vi "Write to File Core.vi"(8 "error in":errorcluster, 10 "File Ref":refnum<file>, 11 "Exe Write CRD RDs in":refnum<class "Exe Write CRD RDs.lvclass">) -> (0 "error out":errorcluster, 3 "Exe Write CRD RDs out":refnum<class "Exe Write CRD RDs.lvclass">)   [LabVIEW 2014, in "Controller.lvlib" / "Exe Write CRD RDs.lvclass"]
uses:
  Exe Write CRD RDs.lvclass
  reusable/Data/Data.lvclass
  Instr Exe Write to File/Instr Exe Write to File.lvclass/Instr Exe Write to File.ctl
  reusable/CRDS/Data/Main/CRDS Data.lvclass
  reusable/CRDS/Data/Cell/CRDS Cell Data.lvclass/CRDS Cell Data.ctl
  reusable/CRDS/Data/Cell/Read Laser Data.vi
  Instr Exe Write to File/Read MAP DVR.vi
  Instr Exe Write to File/Read DataObj.vi
  reusable/Data/Read measTime.vi
  reusable/CRDS/Data/Main/Read CellData.vi
  reusable/CRDS/Data/Cell/CRDS Cell Data.lvclass
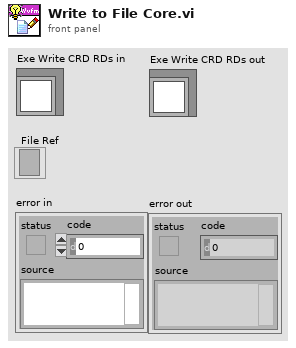
[diagram p1: front panel]
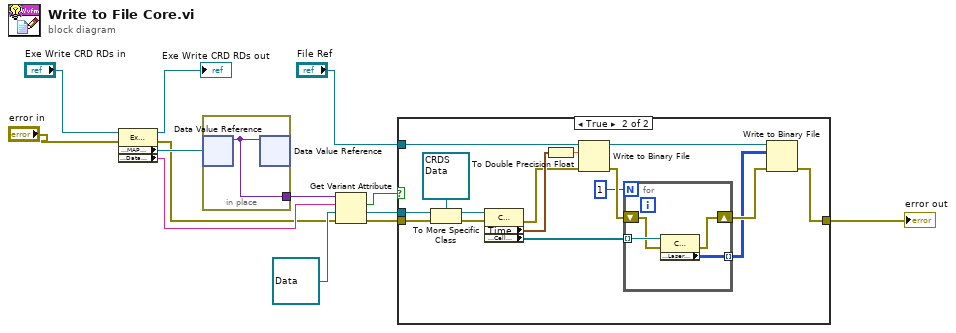
[diagram p0: block diagram]
diagram:
  n1 = property class="Exe Write CRD RDs"(reference="Exe Write CRD RDs in", error in="error in") -> (reference out=→"Exe Write CRD RDs out":refnum<class "Exe Write CRD RDs.lvclass">, error out=w6:errorcluster, "Accessors:MAP DVR"=w9:refnum<data-value>, "Accessors:DataObj"=w8:string)
  n2 = in-place {
    in-place-border: [w14] -> w13
    n3 = in-place-dvr #1(w9) -> (w14:variant)  [unwired: 1 out]
    n4 = in-place-dvr #1(w14) -> ()  [unwired: 2 out]
  }
  n5 = Get Variant Attribute(Variant=w13, name=w8, default value (empty Variant)=refnum<class "Data.lvclass"> refnum ("Base Data Lib:Data"), error in=w6) -> (found=w11:bool, value=w12:refnum<class "Data.lvclass">, error out=w10:errorcluster)  [unwired: 1 out]
  n6 = case shown="True" w11 {
    tunnel: [w15 w18] -> w1
    tunnel: "File Ref" -> [_ w26]
    tunnel: w12 -> [_ w31]
    tunnel: w10 -> [w15 w24]
    frame False {
    }
    frame True {
      n7 = To More Specific Class(target class=refnum<class "CRDS Data.lvclass"> refnum ("CRDS Lib.lvlib:CRDS"), reference=w31, error in=w24) -> (specific class reference=w30:refnum<class "CRDS Data.lvclass">, error out=w23:errorcluster)
      n8 = property class="CRDS"(reference=w30, error in=w23) -> (error out=w22:errorcluster, "Time"=w28:timestamp, "Accessors:Cell Data"=w29:refnum<class "CRDS Cell Data.lvclass">[])  [unwired: 1 out]
      n9 = To Double Precision Float(number=w28) -> (double precision float=w27:dbl)
      n10 = Write to Binary File(file (use dialog)=w26, data=w27, error in=w22) -> (refnum out=w20:refnum<file>, error out=w25:errorcluster)  [unwired: 3 in, 1 out]
      n11 = for {
        N: 1 -> [_]
        tunnel: w29 -> [w35] mode=indexing
        shift-right: [w33] -> w21
        shift-left: w25 -> [w34]
        tunnel: [w32] -> w19 mode=indexing
        n12 = property class="CRDS Cell"(reference=w35, error in=w34) -> (error out=w33:errorcluster, "Accessors:Laser Data"=w32:i16[][])  [unwired: 1 out]
      }
      n13 = Write to Binary File(file (use dialog)=w20, data=w19, error in=w21) -> (error out=w18:errorcluster)  [unwired: 3 in, 2 out]
    }
  }
  "error out" <- w1
